vi "Read ClusDispQueue.vi"(8 "error in (no error)":errorcluster, 11 "DataReceiver in":refnum<class "DataReceiver.lvclass">) -> (0 "error out":errorcluster, 2 "ClusDispQueue":refnum<queue>, 3 "DataReceiver out":refnum<class "DataReceiver.lvclass">)   [LabVIEW 2010, in "DataReceiver.lvclass"]
uses:
  DataReceiver.lvclass
  DataReceiver.lvclass/DataReceiver.ctl
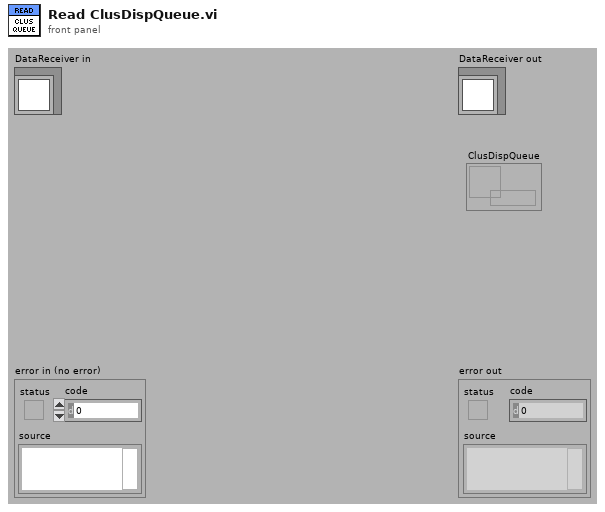
[diagram p1: front panel]
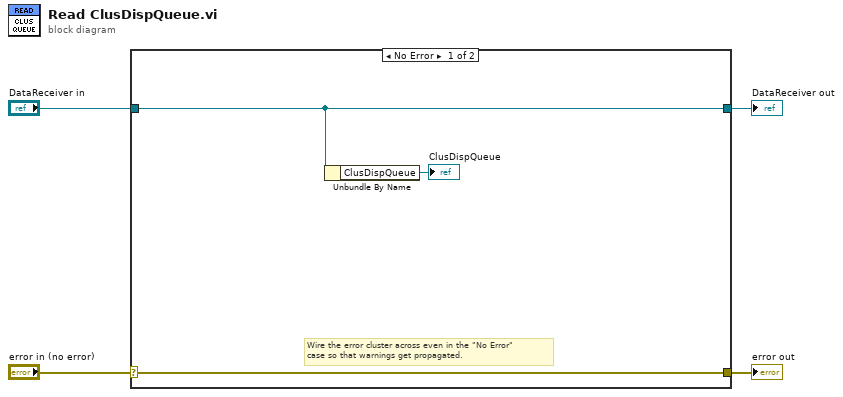
[diagram p0: block diagram]
diagram:
  n1 = case shown="No Error" "error in (no error)" {
    selector: "error in (no error)" -> [w7 w9]
    tunnel: [w7 w9] -> w3
    tunnel: [w6 w8] -> w1
    tunnel: "DataReceiver in" -> [w6 w8]
    frame No Error {
      # "Wire the error cluster across even in the \"No Error\"\ncase so that warnings get propagated."
      n2 = Unbundle By Name(w6) -> ("ClusDispQueue"=→"ClusDispQueue":refnum<queue>)
    }
    frame Error {
    }
  }
  "error out" <- w3
  "DataReceiver out" <- w1
